vi "GPGSV.vi"(10 "String":string, 11 "array":path[](array[path])) -> ()   [LabVIEW 2025]
panel:
  out "size(s) 2":i32
  in  "Selector array":bool[](array[boolean])=[TRUE, TRUE, TRUE, TRUE, TRUE, TRUE, TRUE, TRUE, TRUE, TRUE, TRUE, TRUE, TRUE, TRUE, TRUE, TRUE, TRUE, FALSE, FALSE, FALSE, FALSE, FALSE, TRUE, TRUE, TRUE, TRUE, TRUE, TRUE, TRUE, TRUE, TRUE, TRUE, TRUE, TRUE, TRUE, TRUE, TRUE, FALSE, FALSE, FALSE, FALSE, FALSE, TRUE, TRUE, TRUE, TRUE, TRUE, TRUE, TRUE, FALSE, TRUE]
  out "array w/ subset deleted":string[](array[string])
  out "spreadsheet string":string
  in  "error in":errorcluster
  out "error out 8":errorcluster
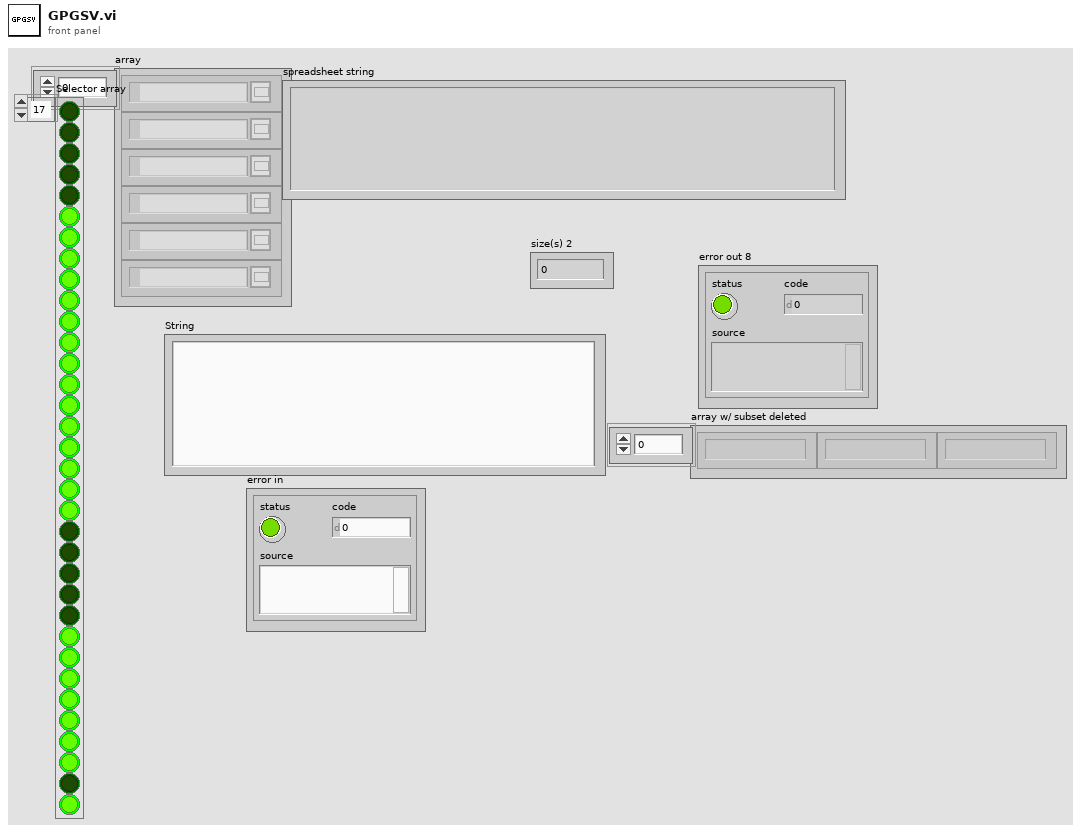
[diagram p1: front panel]
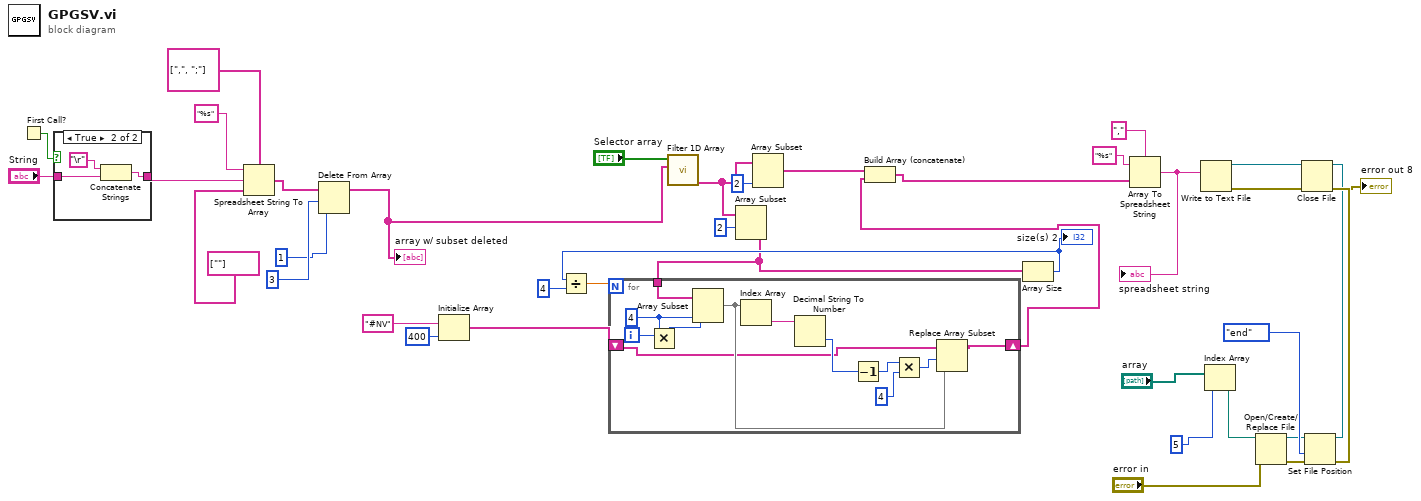
[diagram p0: block diagram]
diagram:
  n1 = First Call?() -> (First Call?: T/F=w25:bool)
  n2 = case shown="True" w25 {
    tunnel: [w40 w42] -> w17
    tunnel: "String" -> [w40 w41]
    frame False {
    }
    frame True {
      n3 = Concatenate Strings("\r", w41) -> (w42:string)
    }
  }
  n4 = Spreadsheet String To Array(delimiter (Tab)=string[] [",", ";"], format string="%s", spreadsheet string=w17, array type (2D Dbl)=string[] [""]) -> (array=w18:string[])
  n5 = Delete From Array(array=w18, length=3, index=1) -> (array with subset deleted=w13:string[])  [unwired: 1 out]
  "array w/ subset deleted" <- w13
  n6 = Initialize Array("#NV" ("element"), 400 ("dimension size")) -> (w7:string[])
  n7 = call "Filter 1D Array.vi"("Input"=w13, "Selector array"="Selector array") -> ("True"=w6:string[])  [unwired: 8 in, 1 out]
  n8 = Array Subset(array=w6, index=2) -> (w8:string[])  [unwired: 1 in]
  n9 = Array Subset(array=w6, length=2) -> (w4:string[])  [unwired: 1 in]
  n10 = Array Size(array=w8) -> (size(s)=w10:i32)
  "size(s) 2" <- w10
  n11 = Divide(x=w10, y=4) -> (x/y=w11:dbl)
  n12 = for {
    N: w11 -> [_]
    tunnel: w8 -> [w55]
    shift-right: [w44] -> w3
    shift-left: w7 -> [w45]
    i -> [w54]
    w52 = 4 ("y")
    n13 = Multiply(x=w54, y=w52) -> (x*y=w53:i32)
    n14 = Array Subset(array=w55, index=w53, length=w52) -> (w46:string[])
    n15 = Index Array(array=w46) -> (element=w48:string)  [unwired: 1 in]
    n16 = Decimal String To Number(string=w48) -> (number=w50:i32)  [unwired: 2 in, 1 out]
    n17 = Decrement(x=w50) -> (x-1=w51:i32)
    n18 = Multiply(x=w51, y=4) -> (x*y=w47:i32)
    n19 = Replace Array Subset(array=w45, new element=w46, index=w47) -> (w44:string[])
  }
  n20 = Build Array (concatenate)(w4, w3) -> (w2:string[])
  n21 = Array To Spreadsheet String(delimiter (Tab)=",", array=w2, 3:"%s" ("format string")) -> (spreadsheet string=w21:string)
  "spreadsheet string" <- w21
  n22 = Index Array(array="array", index=5 ("index (row)")) -> (element=w29:path)
  n23 = Open/Create/Replace File(file path (use dialog)=w29, error in="error in") -> (refnum out=w30:refnum<file>, error out=w33:errorcluster)  [unwired: 4 in, 1 out]
  n24 = Set File Position(refnum=w30, from (0:start)=enum16{"start", "end", "current"}."end", error in=w33) -> (refnum out=w31:refnum<file>, error out=w32:errorcluster)  [unwired: 1 in]
  n25 = Write to Text File(file (use dialog)=w31, text=w21, error in=w32) -> (refnum out=w35:refnum<file>, error out=w34:errorcluster)  [unwired: 1 in, 1 out]
  n26 = Close File(refnum=w35, error in=w34) -> (error out=→"error out 8":errorcluster)  [unwired: 1 out]
